vi "GetMergeMapTb.vi"(1 "FalseColorDat":T2, 2 "VarRangeMin":dbl, 3 "VarRangeMax":dbl) -> (0 "MapTb":T1)   [LabVIEW 2016]
panel:
  # "Description:      This VI is to get  a  false color  mapping table of all  channel (R/G/B)  given real var range(max/min) that you  want to map.\n\nAuthor:               L.F.Hwang  (Email: cn_gd@126.com)\n\nLast Updated:   2007/12/25"
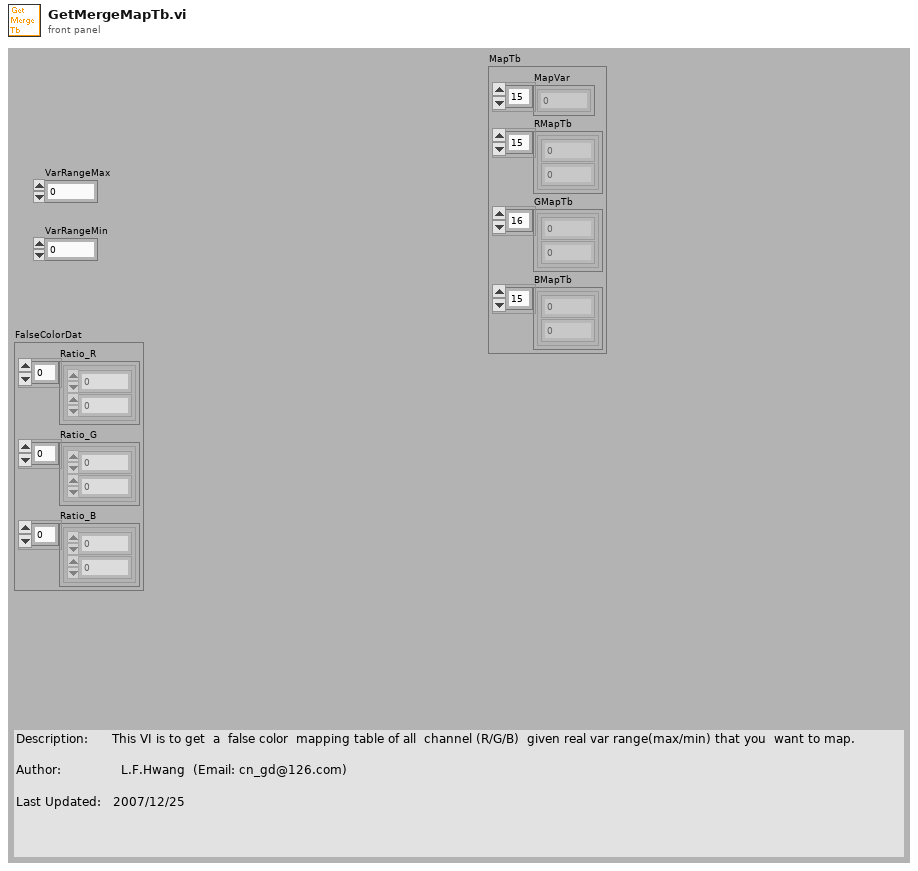
[diagram p1: front panel]
types:
  T1 = cluster{"MapVar":dbl[], "RMapTb":cluster{dbl, u8}[], "GMapTb":cluster{dbl, u8}[], "BMapTb":cluster{dbl, u8}[]}
  T2 = cluster{"Ratio_R":cluster{dbl, dbl}[], "Ratio_G":cluster{dbl, dbl}[], "Ratio_B":cluster{dbl, dbl}[]}
  T3 = cluster{"MapVar":dbl[], "K":dbl[], "RGBValue":u8[]}
  T4 = cluster{dbl[], cluster{dbl, u8}[], cluster{dbl, u8}[], cluster{dbl, u8}[]}
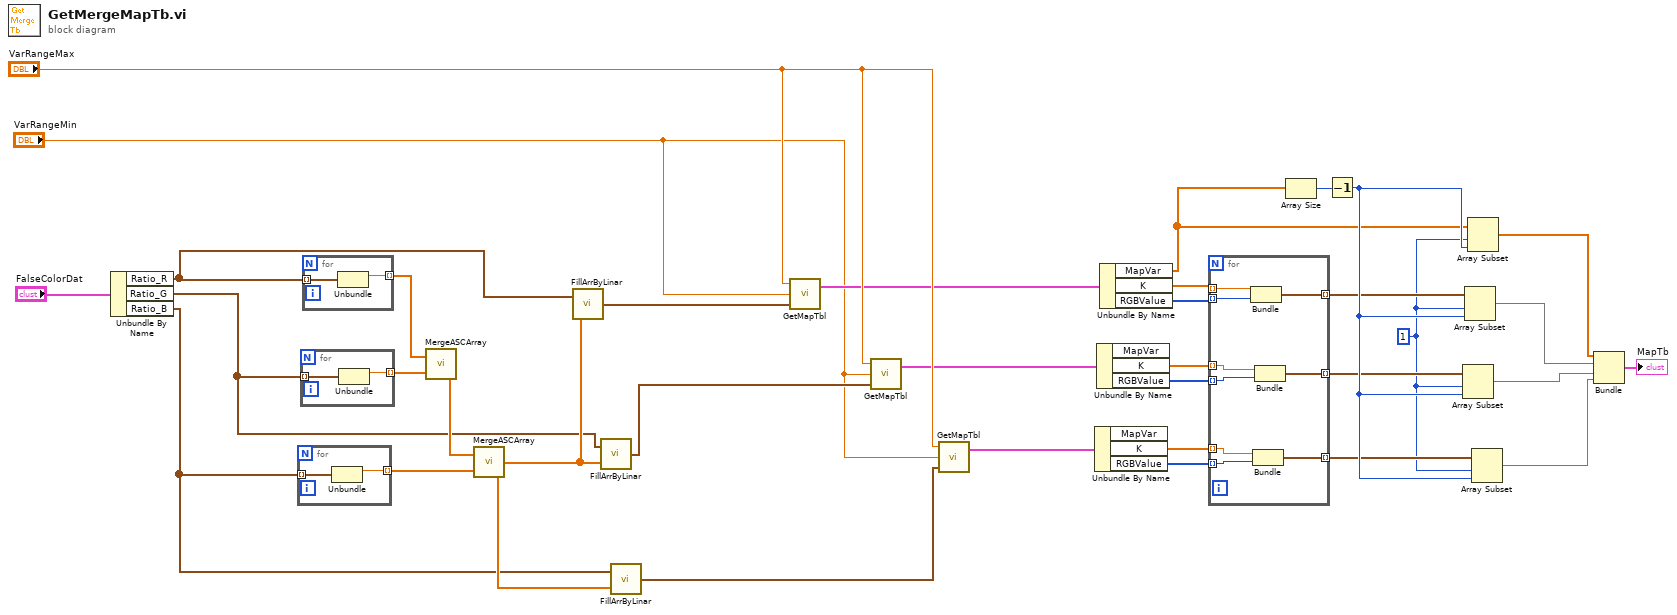
[diagram p0: block diagram]
diagram:
  w3 = 1 ("索引")
  n1 = Unbundle By Name("FalseColorDat") -> ("Ratio_R"=w25:cluster{dbl, dbl}[], "Ratio_G"=w24:cluster{dbl, dbl}[], "Ratio_B"=w23:cluster{dbl, dbl}[])
  n2 = for {
    tunnel: w23 -> [w36] mode=indexing
    tunnel: [w37] -> w26 mode=indexing
    n3 = Unbundle(w36) -> (w37:dbl)  [unwired: 1 out]
  }
  n4 = for {
    tunnel: w24 -> [w39] mode=indexing
    tunnel: [w38] -> w27 mode=indexing
    n5 = Unbundle(w39) -> (w38:dbl)  [unwired: 1 out]
  }
  n6 = for {
    tunnel: w25 -> [w41] mode=indexing
    tunnel: [w40] -> w33 mode=indexing
    n7 = Unbundle(w41) -> (w40:dbl)  [unwired: 1 out]
  }
  n8 = call "MergeASCArray.vi"("Array2"=w27, "Array1"=w33) -> ("Merged Array"=w34:dbl[])
  n9 = call "MergeASCArray.vi"("Array2"=w26, "Array1"=w34) -> ("Merged Array"=w32:dbl[])
  n10 = call "FillArrByLinar.vi"("Filling refence array"=w32, "Cluster Array"=w25) -> ("Filled Cluster Array"=w30:cluster{dbl, dbl}[])
  n11 = call "FillArrByLinar.vi"("Filling refence array"=w32, "Cluster Array"=w24) -> ("Filled Cluster Array"=w29:cluster{dbl, dbl}[])
  n12 = call "FillArrByLinar.vi"("Filling refence array"=w32, "Cluster Array"=w23) -> ("Filled Cluster Array"=w28:cluster{dbl, dbl}[])
  n13 = call "GetMapTbl.vi"("FalseColorDatByCH"=w30, "VarRangeMin"="VarRangeMin", "VarRangeMax"="VarRangeMax") -> ("CHFalseMapTbl"=w22:T3)  [unwired: 1 out]
  n14 = call "GetMapTbl.vi"("FalseColorDatByCH"=w29, "VarRangeMin"="VarRangeMin", "VarRangeMax"="VarRangeMax") -> ("CHFalseMapTbl"=w19:T3)  [unwired: 1 out]
  n15 = call "GetMapTbl.vi"("FalseColorDatByCH"=w28, "VarRangeMin"="VarRangeMin", "VarRangeMax"="VarRangeMax") -> ("CHFalseMapTbl"=w18:T3)  [unwired: 1 out]
  n16 = Unbundle By Name(w18) -> ("K"=w15:dbl[], "RGBValue"=w14:u8[])  [unwired: 1 out]
  n17 = Unbundle By Name(w19) -> ("K"=w17:dbl[], "RGBValue"=w16:u8[])  [unwired: 1 out]
  n18 = Unbundle By Name(w22) -> ("MapVar"=w2:dbl[], "K"=w21:dbl[], "RGBValue"=w20:u8[])
  n19 = for {
    tunnel: w21 -> [w50] mode=indexing
    tunnel: w20 -> [w49] mode=indexing
    tunnel: w17 -> [w48] mode=indexing
    tunnel: w16 -> [w47] mode=indexing
    tunnel: w15 -> [w46] mode=indexing
    tunnel: w14 -> [w45] mode=indexing
    tunnel: [w44] -> w4 mode=indexing
    tunnel: [w43] -> w6 mode=indexing
    tunnel: [w42] -> w8 mode=indexing
    n20 = Bundle(w50, w49) -> (w44:cluster{dbl, u8})  [unwired: 1 out]
    n21 = Bundle(w46, w45) -> (w42:cluster{dbl, u8})  [unwired: 1 out]
    n22 = Bundle(w48, w47) -> (w43:cluster{dbl, u8})  [unwired: 1 out]
  }
  n23 = Array Size(array=w2) -> (size(s)=w11:i32)
  n24 = Decrement(x=w11) -> (x-1=w10:i32)
  n25 = Array Subset(array=w6, index=w3, length=w10) -> (w7:cluster{dbl, u8}[])
  n26 = Array Subset(array=w4, index=w3, length=w10) -> (w5:cluster{dbl, u8}[])
  n27 = Array Subset(array=w2, index=w3, length=w10) -> (w1:dbl[])
  n28 = Array Subset(array=w8, index=w3, length=w10) -> (w9:cluster{dbl, u8}[])
  n29 = Bundle(w1, w5, w7, w9) -> (→"MapTb":T4)  [unwired: 1 out]
